vi "moneda 5.vi"(8 "error in (no error)":errorcluster, 11 "Monedas in":refnum<class "Monedas.lvclass">) -> (0 "error out":errorcluster, 3 "Monedas out":refnum<class "Monedas.lvclass">)   [LabVIEW 2020, in "Monedas.lvlib" / "Monedas.lvclass"]
uses:
  Monedas.lvclass
  C:/Program Files (x86)/National Instruments/LabVIEW 2020/vi.lib/ActorFramework/Actor/Actor.lvclass
  <vilib>/ActorFramework/Actor/Actor.lvclass/Actor.ctl
  Monedas.lvclass/Monedas.ctl
  User Interface Messages/Monedas Msg/Monedas Msg.lvclass/Monedas Msg.ctl
  <vilib>/ActorFramework/Message Enqueuer/Message Enqueuer.lvclass/Message Enqueuer.ctl
  <vilib>/ActorFramework/Message Enqueuer/Enqueue.vi
  User Interface Messages/Monedas Msg/Monedas Msg.lvclass
  C:/Program Files (x86)/National Instruments/LabVIEW 2020/vi.lib/ActorFramework/Message/Message.lvclass
  <vilib>/ActorFramework/Message Priority Queue/Priority Enqueue.vi
  <vilib>/ActorFramework/Actor/Actor.lvclass
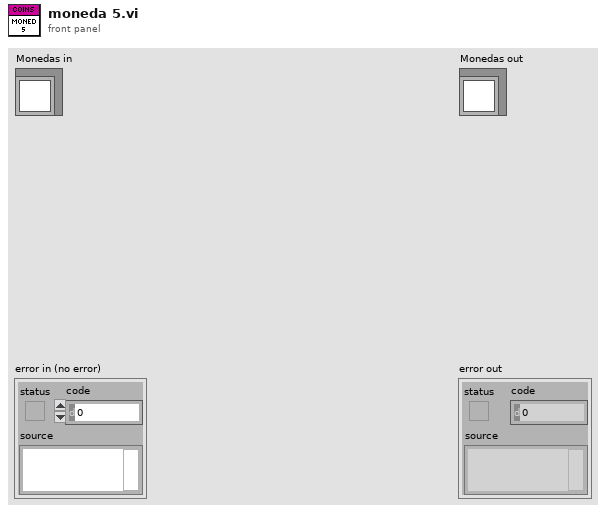
[diagram p1: front panel]
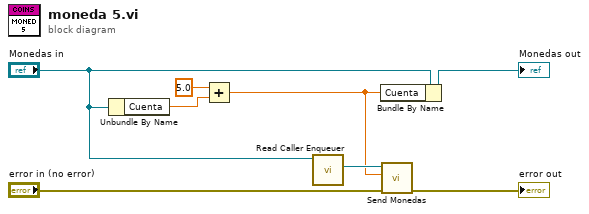
[diagram p0: block diagram]
diagram:
  n1 = Unbundle By Name("Monedas in") -> ("Cuenta"=w7:dbl)
  n2 = Add(x=5.0, y=w7) -> (x+y=w1:dbl)
  n3 = call <vilib>:"Read Caller Enqueuer.vi"("Actor"="Monedas in") -> ("Caller Enqueuer"=w2:refnum<class "Message Enqueuer.lvclass">)  [unwired: 10 in]
  n4 = Bundle By Name(cluster="Monedas in", "Cuenta"=w1) -> (→"Monedas out":refnum<class "Monedas.lvclass">)
  n5 = call "Send Monedas.vi"("error in (no error)"="error in (no error)", "Moneda"=w1, "Message Enqueuer"=w2) -> ("error out"=→"error out":errorcluster)  [unwired: 7 in, 1 out]
